vi "Read Type.vi"(8 "Error In":errorcluster, 11 "Boolean In":refnum<class "Boolean.lvclass">) -> (0 "Error Out":errorcluster, 2 "Type":T1=enum."Boolean", 3 "Boolean Out":refnum<class "Boolean.lvclass">)   [LabVIEW 2018, in "Toolkit.lvlib" / "Data.lvlib" / "Boolean.lvclass"]
doc: "Get the Mustache data type of an object."
uses:
  Boolean.lvclass
  Type Defintions/Types.ctl
  Data.lvlib
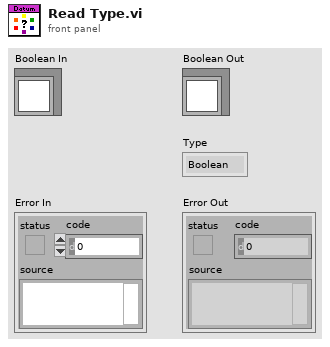
[diagram p1: front panel]
types:
  T1 = typedef "Toolkit.lvlib/Data.lvlib/Types.ctl" = enum16{"Array", "Boolean", "Function", "Map", "Null", "Pair", "Path", "String", "Unknown"}
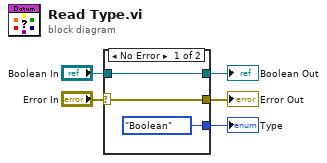
[diagram p0: block diagram]
diagram:
  n1 = case shown="No Error" "Error In" {
    selector: "Error In" -> [w8 w9]
    tunnel: [w8 w9] -> w4
    tunnel: [Types."Boolean" ("Type") _] -> w3
    tunnel: "Boolean In" -> [w6 w10]
    tunnel: [w6 w10] -> w1
    frame No Error {
    }
    frame Error {
    }
  }
  "Error Out" <- w4
  "Boolean Out" <- w1
  "Type" <- w3
